vi "Generate Channels.vi"(8 "error in (no error)":errorcluster, 10 "Type":T2, 11 "Item Ref in":T6 format="%.0x") -> (0 "error out":errorcluster, 1 "Output Channels Out":T1[](array[typedef]) {"Mapping"."VS Reference" format="%.0x"}, 2 "Input Channels Out":T1[](array[typedef]) {"Mapping"."VS Reference" format="%.0x"}, 3 "Item Ref out":T6 format="%.0x")   [LabVIEW 2021, in "Modbus Master System Explorer.lvlib"]
uses:
  Modbus Master System Explorer.lvlib
  Shared/Controls/Data Model/Channel.ctl
  Modbus Type.ctl
  <vilib>/NI VeriStand/Custom Device API/Custom Device Channel Type.ctl
  Shared/Controls/Data Model/Mapping.ctl
  Shared/Controls/Data Model/DataType.ctl
  <vilib>/NI VeriStand/Custom Device API/Custom Device Item Ref.ctl
  <vilib>/NI VeriStand/Custom Device Tools/Custom Device Utility Library/NI VeriStand - Search for Item by GUID.vi
  <vilib>/NI VeriStand/Custom Device Tools/Custom Device Utility Library/Custom Device Utility Library.lvlib
  Shared/Modbus Master Shared.lvlib
  <vilib>/NI VeriStand/Custom Device API/Custom Device API.lvlib
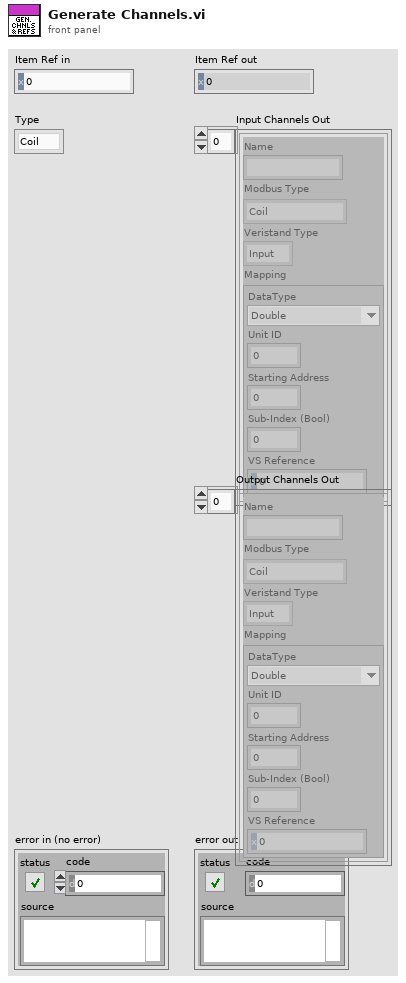
[diagram p1: front panel]
types:
  T1 = typedef "Modbus Master Shared.lvlib/Channel.ctl" = cluster{"Name":string, "Modbus Type":T2, "Veristand Type":T3, "Mapping":T4}
  T2 = typedef "Modbus Master Shared.lvlib/Modbus Type.ctl" = enum16{"Coil", "Discrete Input", "Holding Register", "Input Register"}
  T3 = typedef "Custom Device API.lvlib/Custom Device Channel Type.ctl" = enum16{"Input", "Output"}
  T4 = typedef "Modbus Master Shared.lvlib/Mapping.ctl" = cluster{"DataType":T5, "Unit ID":u8, "Starting Address":u16, "Sub-Index (Bool)":u16, "VS Reference":T6}
  T5 = typedef "Modbus Master Shared.lvlib/DataType.ctl" = enum16{"Double", "Single", "I64", "I32", "I16", "I8", "U64", "U32", "U16", "U8", "Boolean"}
  T6 = typedef "Custom Device API.lvlib/Custom Device Item Ref.ctl" = u64
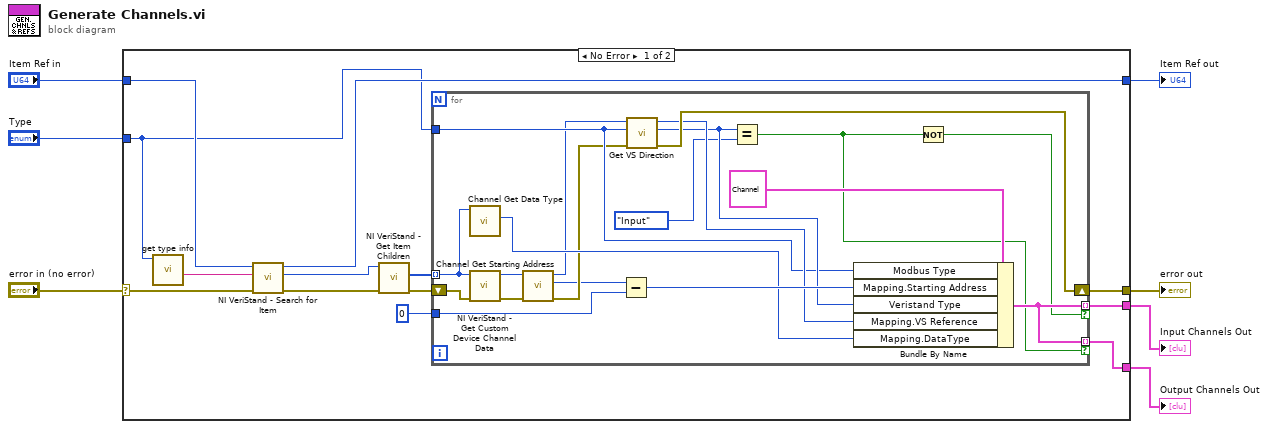
[diagram p0: block diagram]
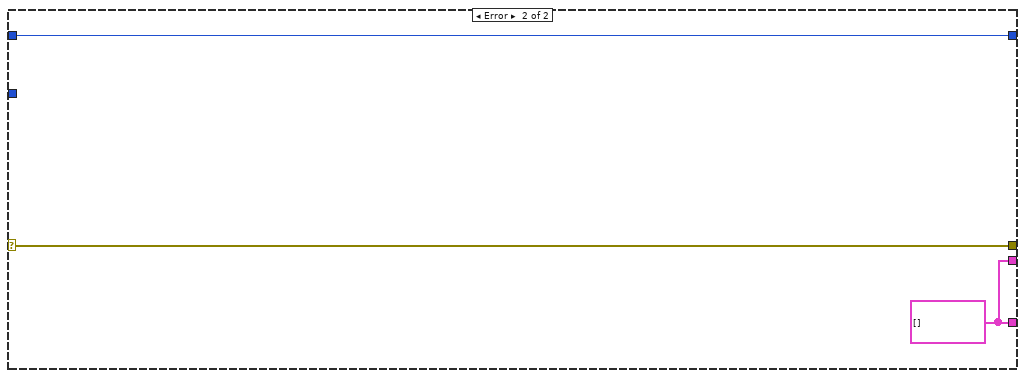
[diagram p2: hidden frame]
diagram:
  n1 = case shown="No Error" "error in (no error)" {
    selector: "error in (no error)" -> [w19 w41]
    tunnel: [w20 w41] -> w7
    tunnel: "Type" -> [w10 _]
    tunnel: "Item Ref in" -> [w18 w42]
    tunnel: [w11 w42] -> w3
    tunnel: [w17 w40] -> w2
    tunnel: [w8 w40] -> w1
    frame No Error {
      n2 = call "get type info.vi"("Type in"=w10) -> ("Group GUID"=w16:string)  [unwired: 8 in, 2 out]
      n3 = call-poly <vilib>:"NI VeriStand - Search for Item.vi"("error in"=w19, "Item GUID"=w16, "Section Ref in"=w18) -> ("error out"=w13:errorcluster, "Item Ref"=w15:T6, "Section Ref out"=w11:T6)  [unwired: 5 in, 1 out]
      n4 = call <vilib>:"NI VeriStand - Get Item Children.vi"("error in (no error)"=w13, "Item Ref in"=w15) -> ("error out"=w12:errorcluster, "Child Refs"=w14:T6[])  [unwired: 6 in, 2 out]
      n5 = for {
        tunnel: w14 -> [w32] mode=indexing
        tunnel: [w29] -> w17 mode=indexing if=w28
        shift-right: [w35] -> w20
        shift-left: w12 -> [w38]
        tunnel: u16 0 ("Offset") -> [w36]
        tunnel: w10 -> [w26]
        tunnel: [w29] -> w8 mode=indexing if=w27
        n6 = call "Channel Get Data Type.vi"("Item Ref in"=w32) -> ("Data Type"=w33:T5)  [unwired: 8 in, 2 out]
        n7 = call <vilib>:"NI VeriStand - Get Custom Device Channel Data.vi"("error in (no error)"=w38, "Channel Ref in"=w32) -> ("error out"=w23:errorcluster, "Channel Ref out"=w25:T6)  [unwired: 4 in, 4 out]
        n8 = call "Channel Get Starting Address.vi"("error in (no error)"=w23, "Item Ref in"=w25) -> ("error out"=w22:errorcluster, "Value"=w21:u16, "Item Ref out"=w24:T6)  [unwired: 7 in]
        n9 = Subtract(x=w21, y=w36) -> (x-y=w37:u16)
        n10 = call "Get VS Direction.vi"("error in (no error)"=w22, "Modbus Type"=w26, "Item Ref in"=w24) -> ("error out"=w35:errorcluster, "Veristand Type"=w31:T3, "Item Ref out"=w34:T6)  [unwired: 6 in]
        n11 = Equal?(x=w31, y=Custom_Device_Channel_Type."Input") -> (x = y?=w27:bool)
        n12 = Bundle By Name(cluster=T1 {"Name"="", "Modbus Type"=enum."Input Register", "Veristand Type"=enum."Input", "Mapping"={"DataType"=enum."Boolean", "Unit ID"=0, "Starting Address"=0, "Sub-Index (Bool)"=0, "VS Reference"=0}} ("Channel"), "Modbus Type"=w26, "Mapping.Starting Address"=w37, "Veristand Type"=w31, "Mapping.VS Reference"=w34, "Mapping.DataType"=w33) -> (w29:T1)
        n13 = Not(x=w27) -> (.not. x?=w28:bool)
      }
    }
    frame Error {
      w40 = T1[] []
    }
  }
  "error out" <- w7
  "Input Channels Out" <- w2
  "Item Ref out" <- w3
  "Output Channels Out" <- w1
